vi "Msg - Receive Module Data.vi"(11 "error in (no error)":errorcluster) -> (4 "Module Data Out":T1, 15 "error out":errorcluster)   [LabVIEW 2016, in "Error Handler - Logger.lvlib"]
doc: "Allows controller to receive the Module Data of THIS Module"
uses:
  Error Handler - Logger.lvlib
  Controls/Module - Data.ctl
  Modules.ctl
  Controls/Module - States.ctl
  Controls/Timing - Data.ctl
  Controls/Process - Element.ctl
  Controls/Process.ctl
  Controls/Process - Status.ctl
  Controls/Current Error Details.ctl
  Controls/Error Types.ctl
  Controls/Message - Queue Manager Mode.ctl
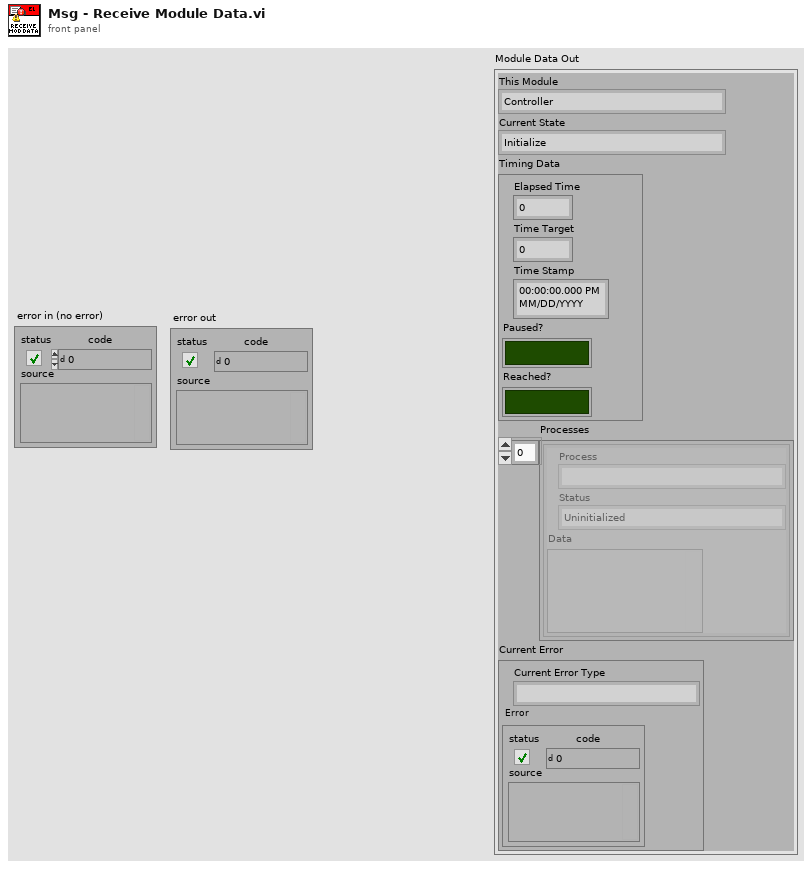
[diagram p1: front panel]
types:
  T1 = typedef "Error Handler - Logger.lvlib/Module - Data.ctl" = cluster{"This Module":T2, "Current State":T3, "Timing Data":T4, "Processes":T5[], "Current Error":T8}
  T2 = typedef "Error Handler - Logger.lvlib/Modules.ctl" = enum16{"Controller", "Error Handler - Logger"}
  T3 = typedef "Error Handler - Logger.lvlib/Module - States.ctl" = enum16{"Initialize", "Event ", "Send data", "FP Element: Update", "FP Element: Disable/Enable", "Timer: Setup", "Terminate", "--------Template----------", "Process Error", "Log ", "Log Error"}
  T4 = typedef "Error Handler - Logger.lvlib/Timing - Data.ctl" = cluster{"Elapsed Time":dbl, "Time Target":dbl, "Time Stamp":timestamp, "Paused?":bool, "Reached?":bool}
  T5 = typedef "Error Handler - Logger.lvlib/Process - Element.ctl" = cluster{"Process":T6, "Status":T7, "Data":variant}
  T6 = typedef "Error Handler - Logger.lvlib/Process.ctl" = enum16{""}
  T7 = typedef "Error Handler - Logger.lvlib/Process - Status.ctl" = enum16{"Uninitialized", "Busy"}
  T8 = typedef "Error Handler - Logger.lvlib/Current Error Details.ctl" = cluster{"Current Error Type":T9, "Error":errorcluster}
  T9 = typedef "Error Handler - Logger.lvlib/Error Types.ctl" = enum16{""}
  T10 = typedef "Error Handler - Logger.lvlib/Message - Queue Manager Mode.ctl" = enum16{"Create", "Get", "Destroy"}
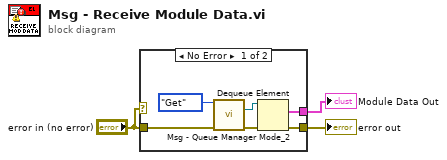
[diagram p0: block diagram]
diagram:
  n1 = case shown="No Error" "error in (no error)" {
    tunnel: [w6 _] -> w3
    tunnel: [w4 w10] -> w2
    tunnel: "error in (no error)" -> [w5 w10]
    frame No Error {
      n2 = call "Msg - Queue Manager Mode_2.vi"("Mode"=Message_-_Queue_Manager_Mode."Get", "error in (no error)"=w5) -> (">>Controller"=w7:refnum<queue>, "error out"=w8:errorcluster)  [unwired: 11 in, 1 out]
      n3 = Dequeue Element(queue=w7, error in (no error)=w8) -> (element=w6:T1, error out=w4:errorcluster)  [unwired: 1 in, 2 out]
    }
    frame Error {
    }
  }
  "error out" <- w2
  "Module Data Out" <- w3
